vi "DAQ Port1 State - Read.vi"(8 "error in":errorcluster, 11 "TSM Context Global Access in":refnum<class "TSM Context Data Access.lvclass">) -> (0 "error out":errorcluster, 2 "DAQ Port1 State":bool[](array[boolean]), 3 "TSM Context Global Access out":refnum<class "TSM Context Data Access.lvclass">)   [LabVIEW 2019, in "TSM Context Data Access.lvclass"]
uses:
  TSM Context Data Access.lvclass
  TSM Context Data Access.lvclass/TSM Context Data Access.ctl
  <vilib>/NI_TestStand_SemiconductorModule/NI_TestStand_Semiconductor_Module.lvlibp
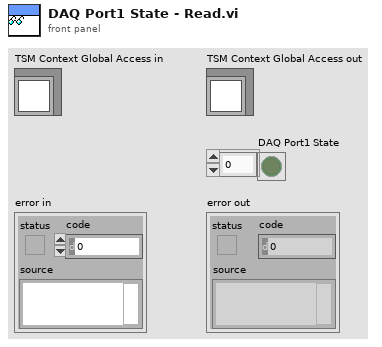
[diagram p1: front panel]
types:
  T1 = typedef "NI_TestStand_Semiconductor_Module.lvlibp/SemiconductorModuleContext.ctl" = refnum<k7>
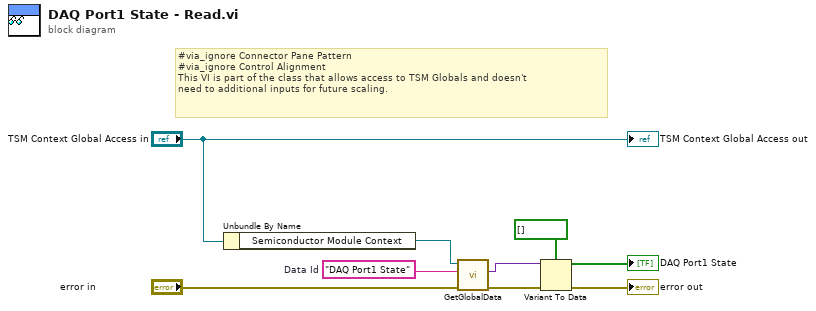
[diagram p0: block diagram]
diagram:
  w4 = "DAQ Port1 State"  # Data Id
  # "#via_ignore Connector Pane Pattern\n#via_ignore Control Alignment \nThis VI is part of the class that allows access to TSM Globals and doesn't \nneed to additional inputs for future scaling."
  n1 = Unbundle By Name("TSM Context Global Access in") -> ("Semiconductor Module Context"=w3:T1)
  n2 = call <vilib>:"GetGlobalData.vi"("error in (no error)"="error in", "Data Id"=w4, "Semiconductor Module Context"=w3) -> ("error out"=w5:errorcluster, "Data"=w2:variant)  [unwired: 6 in, 1 out]
  n3 = Variant To Data(error in=w5, type=bool[] [], Variant=w2) -> (data=→"DAQ Port1 State":bool[], error out=→"error out":errorcluster)
  "TSM Context Global Access out" <- "TSM Context Global Access in"
